vi "Add Null Terminator.vi"(5 "New Wifi Config in":T1) -> (2 "New Wifi Config out":T1)   [LabVIEW 2019, in "LINXx.lvlib"]
doc: "Adds null character (\\0) to end of strings in WiFi settings."
uses:
  <vilib>/MakerHub/LINX/Private/Device/Type Defs/Wifi Config.ctl
  <vilib>/MakerHub/LINX/Private/Type Defs/WIFI Security Type.ctl
  LINXx.lvlib
  <vilib>/MakerHub/LINX/LMH-LINX.lvlib
  <vilib>/MakerHub/LINX/Private/Device/Device.lvlib
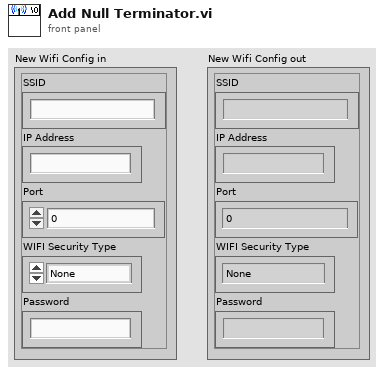
[diagram p1: front panel]
types:
  T1 = typedef "LMH-LINX.lvlib/Device.lvlib/Wifi Config.ctl" = cluster{"SSID":string, "IP Address":string, "Port":u16, "WIFI Security Type":T2, "Password":string}
  T2 = typedef "LMH-LINX.lvlib/WIFI Security Type.ctl" = enum8{"None", "WPA2 Password", "WPA2 Key", "WEP40", "WEP104"}
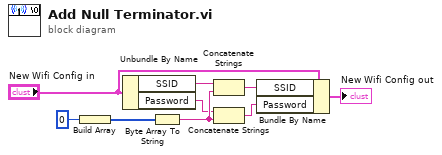
[diagram p0: block diagram]
diagram:
  n1 = Build Array(u8 0) -> (w4:u8[])
  n2 = Unbundle By Name("New Wifi Config in") -> ("SSID"=w7:string, "Password"=w2:string)
  n3 = Byte Array To String(unsigned byte array=w4) -> (string=w8:string)
  n4 = Concatenate Strings(w7, w8) -> (w5:string)
  n5 = Concatenate Strings(w2, w8) -> (w6:string)
  n6 = Bundle By Name(cluster="New Wifi Config in", "SSID"=w5, "Password"=w6) -> (→"New Wifi Config out":T1)
